vi "启动参数显隐控制.vi"(8 "error in (no error)":errorcluster, 11 "控件":refnum<vi>) -> (0 "error out":errorcluster)   [LabVIEW 2016]
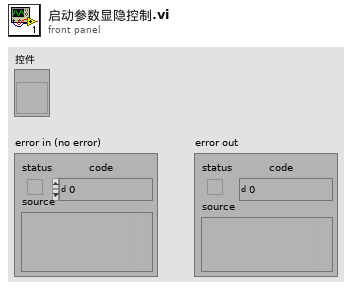
[diagram p1: front panel]
types:
  T1 = typedef "启动参数.ctl" = cluster{"氨氮":bool, "总磷":bool, "总氮":bool, "多参数":bool, "CODmn":bool, "CODCr":bool, "氟化物":bool, "超标留样":bool, "重金属":bool, "挥发酚":bool}
  T2 = typedef "模块配置类型.ctl" = enum16{"单模块", "总磷总氮二合一模块", "氨氮总磷二合一模块"}
  T3 = cluster{"[0]":bool, "[1]":bool, "[2]":bool, "[3]":bool, "[4]":bool, "[5]":bool, "[6]":bool, "[7]":bool, "[8]":bool, "[9]":bool}
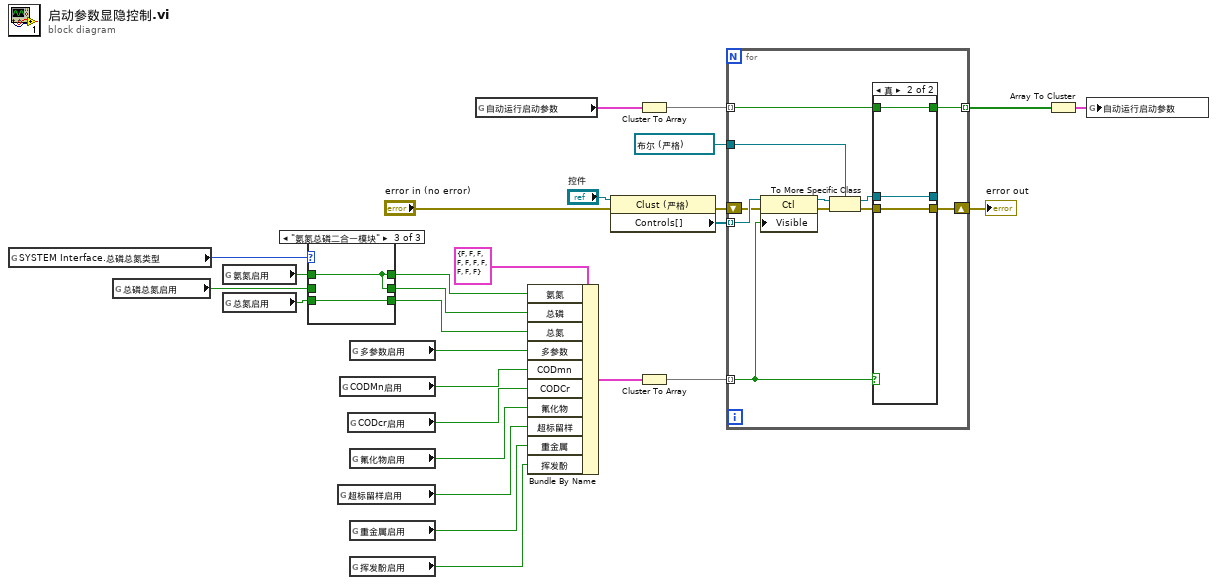
[diagram p0: block diagram]
diagram:
  n1 = global read "系统设置全局变量.vi" "SYSTEM Interface.总磷总氮类型"() -> (w11:T2)
  n2 = global read "系统设置全局变量.vi" "总磷总氮启用"() -> (w8:bool)
  n3 = global read "系统设置全局变量.vi" "氨氮启用"() -> (w10:bool)
  n4 = global read "系统设置全局变量.vi" "总氮启用"() -> (w9:bool)
  n5 = case shown="\"氨氮总磷二合一模块\"" w11 {
    tunnel: [w28 w32 w34] -> w7
    tunnel: [w29 w32 w33] -> w6
    tunnel: [w30 w31 w34] -> w5
    tunnel: w10 -> [w30 w31 w34]
    tunnel: w9 -> [w29 _ w33]
    tunnel: w8 -> [w28 w32 _]
    frame "单模块", Default {
    }
    frame "总磷总氮二合一模块" {
    }
    frame "氨氮总磷二合一模块" {
    }
  }
  n6 = global read "系统设置全局变量.vi" "超标留样启用"() -> (w21:bool)
  n7 = global read "系统设置全局变量.vi" "CODMn启用"() -> (w19:bool)
  n8 = global read "系统设置全局变量.vi" "CODcr启用"() -> (w16:bool)
  n9 = global read "系统设置全局变量.vi" "多参数启用"() -> (w18:bool)
  n10 = global read "系统设置全局变量.vi" "氟化物启用"() -> (w20:bool)
  n11 = global read "系统设置全局变量.vi" "重金属启用"() -> (w17:bool)
  n12 = global read "系统设置全局变量.vi" "挥发酚启用"() -> (w15:bool)
  n13 = global read "系统设置全局变量.vi" "自动运行启动参数"() -> (w4:T1)
  n14 = Bundle By Name(cluster=T1 {"氨氮"=FALSE, "总磷"=FALSE, "总氮"=FALSE, "多参数"=FALSE, "CODmn"=FALSE, "CODCr"=FALSE, "氟化物"=FALSE, "超标留样"=FALSE, "重金属"=FALSE, "挥发酚"=FALSE} ("显隐设置"), "氨氮"=w5, "总磷"=w7, "总氮"=w6, "多参数"=w18, "CODmn"=w19, "CODCr"=w16, "氟化物"=w20, "超标留样"=w21, "重金属"=w17, "挥发酚"=w15) -> (w22:T1)
  n15 = property class="Clust (严格)"(reference="控件", error in="error in (no error)") -> (error out=w14:errorcluster, "Controls[]"=w24:refnum<vi>[])  [unwired: 1 out]
  n16 = Cluster To Array(cluster=w4) -> (array=w3:bool[])
  n17 = Cluster To Array(cluster=w22) -> (array=w26:bool[])
  n18 = for {
    tunnel: w24 -> [w45] mode=indexing
    tunnel: w26 -> [w40] mode=indexing
    tunnel: refnum<vi> refnum ("氨氮") -> [w42]
    shift-right: [w35] -> w13
    shift-left: w14 -> [w39]
    tunnel: w3 -> [w37] mode=indexing
    tunnel: [w36] -> w2 mode=indexing
    n19 = property class="Ctl"(reference=w45, error in=w39, "Visible"=w40) -> (reference out=w44:refnum<vi>, error out=w43:errorcluster)
    n20 = To More Specific Class(target class=w42, reference=w44, error in=w43) -> (specific class reference=w41:refnum<vi>, error out=w38:errorcluster)
    n21 = case shown="真" w40 {
      tunnel: w41 -> [w47 w50]
      tunnel: [w47 w50] -> _
      tunnel: [w46 w49] -> w35
      tunnel: w38 -> [w46 w49]
      tunnel: w37 -> [_ w48]
      tunnel: [_ w48] -> w36
      frame False {
      }
      frame True {
      }
    }
  }
  "error out" <- w13
  n22 = Array To Cluster(array=w2) -> (cluster=w1:T3)
  n23 = global write "系统设置全局变量.vi" "自动运行启动参数"(w1) -> ()
